vi "2. Tutorials.vi"() -> ()   [LabVIEW 2019]
uses:
  <vilib>/Platform/browser.llb/Open URL in Default Browser (string).vi
panel:
  in  "Video options":i32(listbox)
  # "Going to the URL"
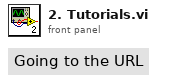
[diagram p1: front panel]
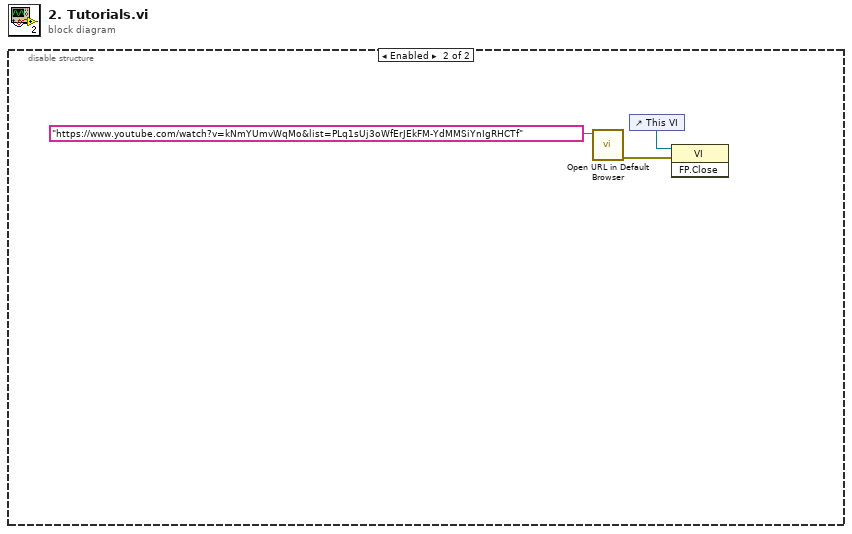
[diagram p0: block diagram]
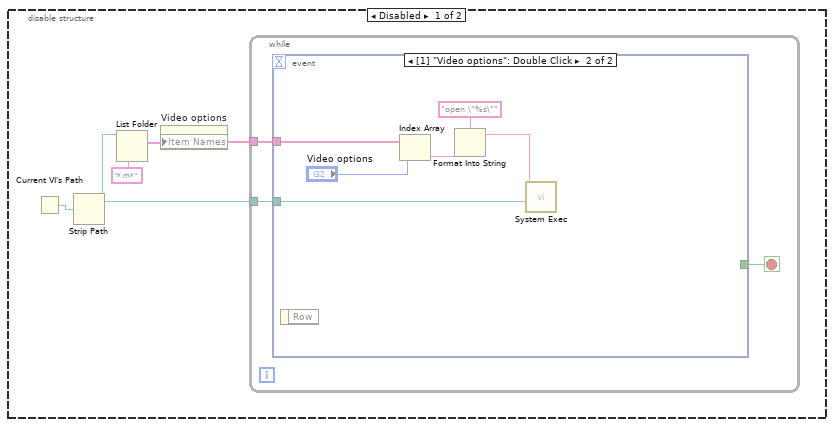
[diagram p2: hidden frame]
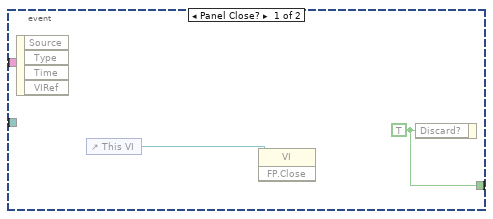
[diagram p3: hidden frame]
diagram:
  n1 = disable-structure shown="Enabled" {
    frame Disabled {
      n2 = Current VI's Path() -> (path=w4:path)
      n3 = Strip Path(path=w4) -> (stripped path=w1:path)  [unwired: 1 out]
      n4 = List Folder(path=w1, pattern="*.m*") -> (filenames=w2:string[])  [unwired: 2 in, 3 out]
      n5 = property on="Video options" class="LstBox (strict)"("Item Names"=w2) -> ()  [unwired: 2 in, 2 out]
      n6 = while {
        tunnel: w2 -> [w6]
        tunnel: w1 -> [w5]
        stop <- w7 stop-if-true
        n7 = event shown="[1] \"Video options\": Double Click" {
          selector: _ -> [_ _]
          dyn-events: _ -> [_ _]
          timeout: _ -> [_ _]
          tunnel: [w9 _] -> w7
          tunnel: w6 -> [_ w15]
          tunnel: w5 -> [_ w11]
          event Panel Close? {
            w9 = TRUE ("Discard?")
            n8 = event-data() -> ()  [unwired: 1 in, 4 out]
            n9 = control-ref of="This VI"() -> (w8:refnum<vi>)
            n10 = invoke class="VI" method="FP.Close"(reference=w8) -> ()  [unwired: 2 in, 3 out]
            n11 = event-data("Discard?"=w9) -> ()  [unwired: 1 in, 1 out]
          }
          event "Video options": Double Click {
            n12 = event-data() -> ()  [unwired: 1 in, 1 out]
            n13 = Index Array(array=w15, index="Video options") -> (element=w10:string)
            n14 = Format Into String(format string="open \"%s\"", w10) -> (resulting string=w12:string)  [unwired: 2 in, 1 out]
            n15 = call <vilib>:"System Exec.vi"("working directory"=w11, "command line"=w12) -> ()  [unwired: 6 in, 4 out]
          }
        }
      }
    }
    frame Enabled {
      n16 = call-poly <vilib>:"Open URL in Default Browser.vi"("URL"="https://www.youtube.com/watch?v=kNmYUmvWqMo&list=PLq1sUj3oWfErJEkFM-YdMMSiYnIgRHCTf") -> ("error out"=w16:errorcluster)  [unwired: 5 in, 1 out]
      n17 = control-ref of="This VI"() -> (w17:refnum<vi>)
      n18 = invoke class="VI" method="FP.Close"(reference=w17, error in=w16) -> ()  [unwired: 1 in, 3 out]
    }
  }
